vi "Loop Get ShiftRegister Input Output Assignements VHDL.vi"(10 "Inside Terms[] offset 2":i32, 11 "RightShiftRegister[]":refnum<vi>[](array[refnum])) -> (0 "right shift regs outside wires assgn.":string, 1 "init values":string, 2 "output assignements":string, 3 "input assignements":string)   [LabVIEW 2018]
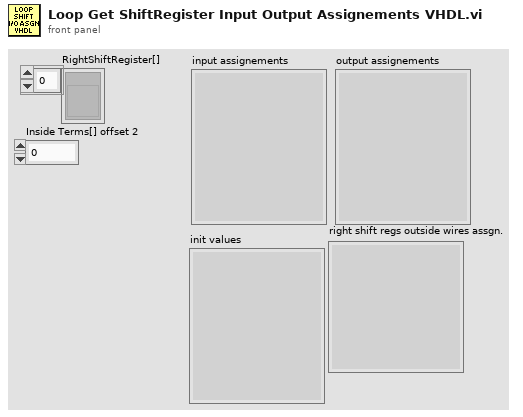
[diagram p1: front panel]
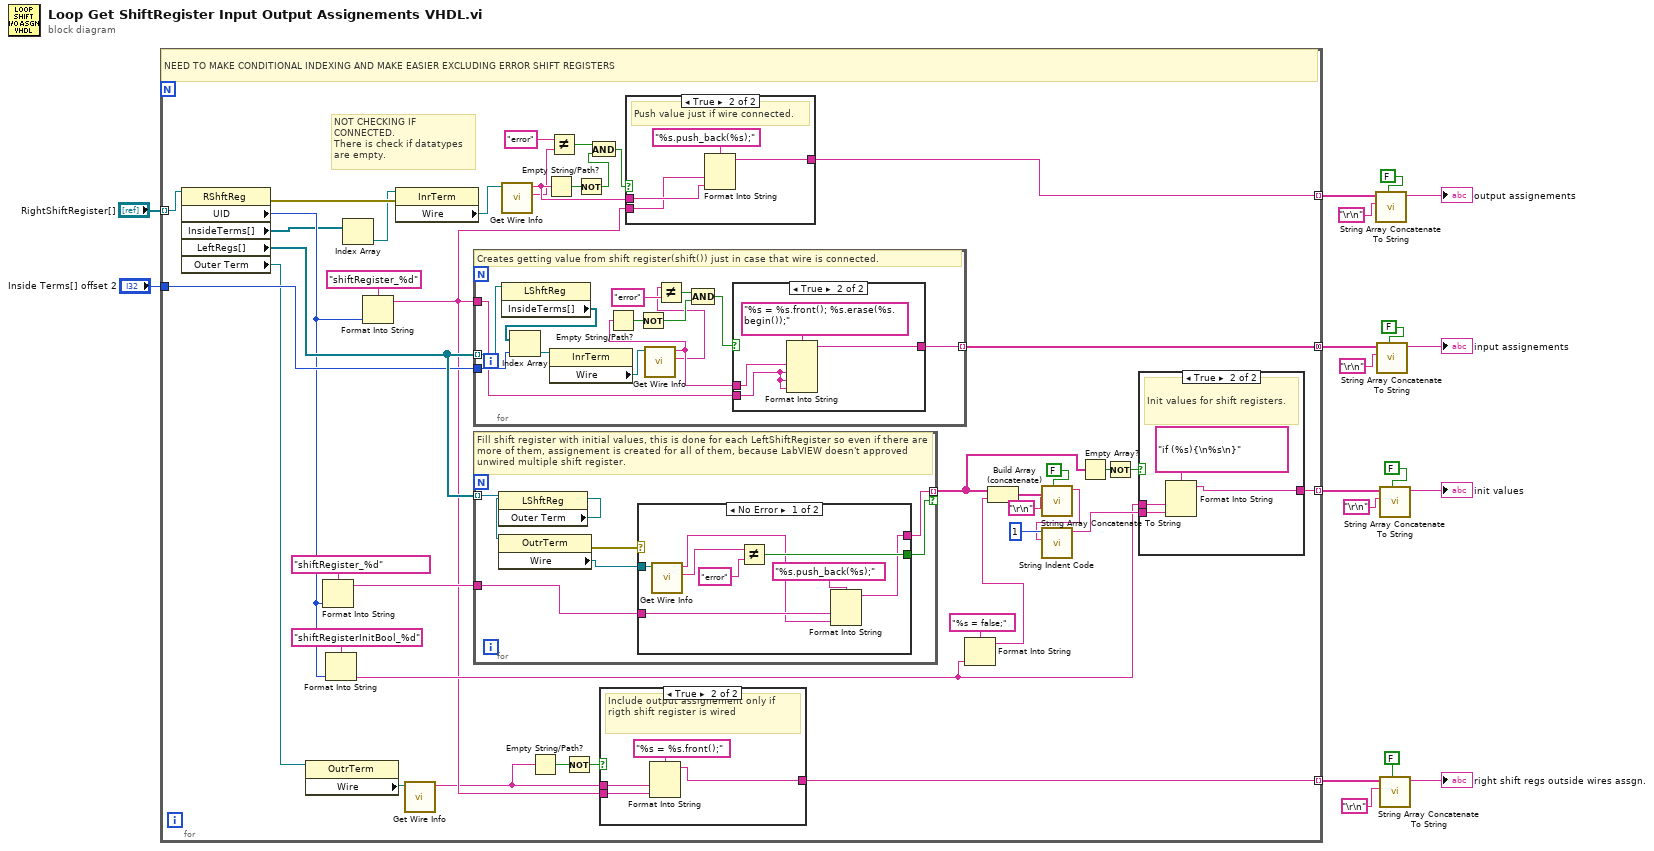
[diagram p0: block diagram]
diagram:
  n1 = for {
    tunnel: "RightShiftRegister[]" -> [w58] mode=indexing
    tunnel: "Inside Terms[] offset 2" -> [w42]
    tunnel: [w55] -> w10 mode=concatenating
    tunnel: [w52] -> w11 mode=indexing
    tunnel: [w41] -> w5 mode=indexing
    tunnel: [w22] -> w2 mode=indexing
    # "NOT CHECKING IF CONNECTED.\nThere is check if datatypes are empty."
    # "NEED TO MAKE CONDITIONAL INDEXING AND MAKE EASIER EXCLUDING ERROR SHIFT REGISTERS"
    n2 = property class="RShftReg"(reference=w58) -> (error out=w59:errorcluster, "UID"=w33:i32, "InsideTerms[]"=w27:refnum<vi>[], "LeftRegs[]"=w46:refnum<vi>[], "Outer Term"=w25:refnum<vi>)  [unwired: 1 in, 1 out]
    n3 = property class="OutrTerm"(reference=w25) -> ("Wire"=w24:refnum<vi>)  [unwired: 1 in, 2 out]
    n4 = Format Into String(format string="shiftRegister_%d", w33) -> (resulting string=w31:string)  [unwired: 2 in, 1 out]
    n5 = Format Into String(format string="shiftRegisterInitBool_%d", w33) -> (resulting string=w29:string)  [unwired: 2 in, 1 out]
    n6 = Index Array(array=w27) -> (element=w26:refnum<vi>)  [unwired: 1 in]
    n7 = Format Into String(format string="shiftRegister_%d", w33) -> (resulting string=w23:string)  [unwired: 2 in, 1 out]
    n8 = property class="InrTerm"(reference=w26, error in=w59) -> ("Wire"=w57:refnum<vi>)  [unwired: 2 out]
    n9 = call "Get Wire Info.vi"("Wire"=w24) -> ("wire label"=w20:string)  [unwired: 9 in, 1 out]
    n10 = for {
      tunnel: w42 -> [w97]
      tunnel: w46 -> [w94] mode=indexing
      tunnel: w23 -> [w90]
      tunnel: [w88] -> w55 mode=indexing
      # "Creates getting value from shift register(shift()) just in case that wire is connected."
      n11 = property class="LShftReg"(reference=w94) -> ("InsideTerms[]"=w93:refnum<vi>[])  [unwired: 1 in, 2 out]
      n12 = Index Array(array=w93, index=w97) -> (element=w92:refnum<vi>)
      n13 = property class="InrTerm"(reference=w92) -> ("Wire"=w100:refnum<vi>)  [unwired: 1 in, 2 out]
      n14 = call "Get Wire Info.vi"("Wire"=w100) -> ("wire datatype"=w87:string, "wire label"=w89:string)  [unwired: 9 in]
      n15 = Empty String/Path?(string/path=w89) -> (empty?=w96:bool)
      n16 = Not(x=w96) -> (.not. x?=w95:bool)
      n17 = Not Equal?(x=w87, y="error") -> (x != y?=w99:bool)
      n18 = Compound Arithmetic op=AND(w99, w95) -> (w91:bool)
      n19 = case shown="True" w91 {
        tunnel: w90 -> [_ w101]
        tunnel: w89 -> [_ w103]
        tunnel: [_ w102] -> w88
        frame False {
        }
        frame True {
          n20 = Format Into String(format string="%s = %s.front(); %s.erase(%s.begin());", w103, w101, w101, w101) -> (resulting string=w102:string)  [unwired: 2 in, 1 out]
        }
      }
    }
    n21 = for {
      tunnel: w46 -> [w74] mode=indexing
      tunnel: [w70] -> w34 mode=indexing if=w69
      tunnel: w31 -> [w68]
      # "Fill shift register with initial values, this is done for each LeftShiftRegister so even if there are more of them, assignement is created for all of them, because LabVIEW doesn't approved unwired multiple shift register."
      n22 = property class="LShftReg"(reference=w74) -> ("Outer Term"=w73:refnum<vi>)  [unwired: 1 in, 2 out]
      n23 = property class="OutrTerm"(reference=w73) -> (error out=w71:errorcluster, "Wire"=w72:refnum<vi>)  [unwired: 1 in, 1 out]
      n24 = case shown="No Error" w71 {
        tunnel: w72 -> [w82 _]
        tunnel: [w80 _] -> w69
        tunnel: [w75 _] -> w70
        tunnel: w68 -> [w77 _]
        frame No Error {
          n25 = call "Get Wire Info.vi"("Wire"=w82) -> ("wire datatype"=w79:string, "wire label"=w76:string)  [unwired: 9 in]
          n26 = Not Equal?(x=w79, y="error") -> (x != y?=w80:bool)
          n27 = Format Into String(format string="%s.push_back(%s);", w77, w76) -> (resulting string=w75:string)  [unwired: 2 in, 1 out]
        }
        frame Error {
        }
      }
    }
    n28 = call "Get Wire Info.vi"("Wire"=w57) -> ("wire datatype"=w48:string, "wire label"=w53:string)  [unwired: 9 in]
    n29 = Empty String/Path?(string/path=w20) -> (empty?=w21:bool)
    n30 = Empty String/Path?(string/path=w53) -> (empty?=w54:bool)
    n31 = Not Equal?(x="error" ("y"), y=w48) -> (x != y?=w50:bool)
    n32 = Not(x=w21) -> (.not. x?=w19:bool)
    n33 = Not(x=w54) -> (.not. x?=w51:bool)
    n34 = And(x=w50, y=w51) -> (x .and. y?=w47:bool)
    n35 = case shown="True" w19 {
      tunnel: w20 -> [_ w62]
      tunnel: w23 -> [_ w61]
      tunnel: [_ w60] -> w22
      frame False {
      }
      frame True {
        # "Include output assignement only if rigth shift register is wired"
        n36 = Format Into String(format string="%s = %s.front();", w62, w61) -> (resulting string=w60:string)  [unwired: 2 in, 1 out]
      }
    }
    n37 = case shown="True" w47 {
      tunnel: w23 -> [_ w83]
      tunnel: w53 -> [_ w84]
      tunnel: [_ w85] -> w52
      frame False {
      }
      frame True {
        # "Push value just if wire connected."
        n38 = Format Into String(format string="%s.push_back(%s);", w83, w84) -> (resulting string=w85:string)  [unwired: 2 in, 1 out]
      }
    }
    n39 = Format Into String(format string="%s = false;", w29) -> (resulting string=w28:string)  [unwired: 2 in, 1 out]
    n40 = Build Array (concatenate)(w34, w28) -> (w39:string[])
    n41 = call "String Array Concatenate To String.vi"("insert last delimiter?"=FALSE, "Delimiter char"="\r\n", "Array String In"=w39) -> ("String"=w37:string)  [unwired: 8 in]
    n42 = call "String Indent Code.vi"("complete code"=w37, "actual nested level"=1) -> ("indented code"=w36:string)  [unwired: 9 in]
    n43 = Empty Array?(array=w34) -> (empty?=w35:bool)
    n44 = Not(x=w35) -> (.not. x?=w40:bool)
    n45 = case shown="True" w40 {
      tunnel: w29 -> [_ w66]
      tunnel: w36 -> [_ w65]
      tunnel: [_ w64] -> w41
      frame False {
        # "Remove error shift registers."
      }
      frame True {
        # "Init values for shift registers."
        n46 = Format Into String(format string="if (%s){\n%s\n}", w66, w65) -> (resulting string=w64:string)  [unwired: 2 in, 1 out]
      }
    }
  }
  n47 = call "String Array Concatenate To String.vi"("insert last delimiter?"=FALSE, "Delimiter char"="\r\n", "Array String In"=w11) -> ("String"=→"output assignements":string)  [unwired: 8 in]
  n48 = call "String Array Concatenate To String.vi"("insert last delimiter?"=FALSE, "Delimiter char"="\r\n", "Array String In"=w10) -> ("String"=→"input assignements":string)  [unwired: 8 in]
  n49 = call "String Array Concatenate To String.vi"("insert last delimiter?"=FALSE, "Delimiter char"="\r\n", "Array String In"=w5) -> ("String"=→"init values":string)  [unwired: 8 in]
  n50 = call "String Array Concatenate To String.vi"("insert last delimiter?"=FALSE, "Delimiter char"="\r\n", "Array String In"=w2) -> ("String"=→"right shift regs outside wires assgn.":string)  [unwired: 8 in]
